vi "Handle String Data.vi"(7 "Source ID":u32, 8 "StringData":T1, 9 "Sequence":u32, 10 "ChannelService":refnum<class "ChannelService.lvclass">, 11 "Subscription Loop Data in":T2) -> (0 "error out":errorcluster, 3 "Subscription Loop Data":T2)   [LabVIEW 2020, in "Vecto.lvlib" / "RemoteDataService.lvclass"]
uses:
  RemoteDataService.lvclass
  Subscription Loop Data.ctl
  Subscription Group Info.ctl
  Group/Group.lvclass
  SubscribedDataHandler/SubscribedDataHandler.lvclass
  proto/StringData/Data.ctl
  ChannelService/ChannelService.lvclass
  <vilib>/Utility/miscctls.llb/LVMapReplaceAction.ctl
  Group STR/Group STR.lvclass
  C:/dev/lv20CE/relink/lv-vecto/Vecto/Group/Group.lvclass
  Vecto.lvlib
  proto/StringData/StringData.lvlib
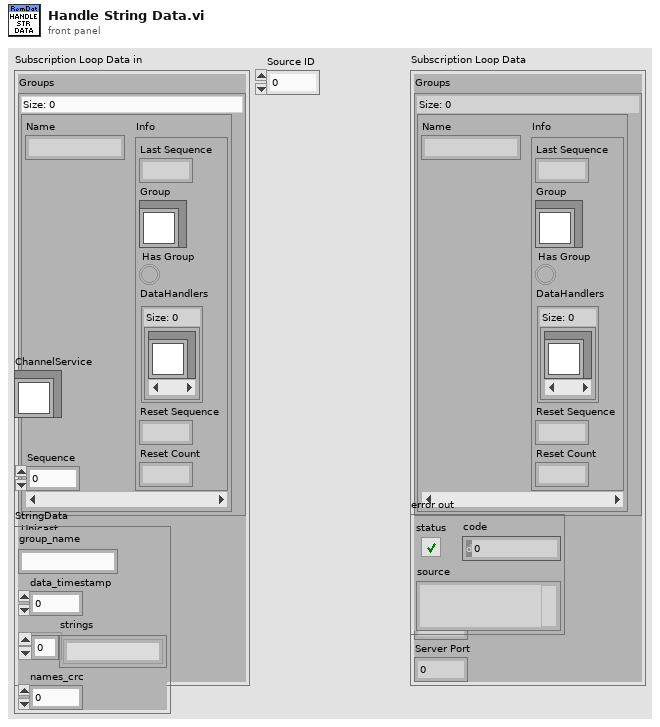
[diagram p1: front panel]
types:
  T1 = typedef "StringData.lvlib/Data.ctl" = cluster{"group_name":string, "data_timestamp":i64, "strings":string[], "names_crc":u32}
  T2 = typedef "Vecto.lvlib/RemoteDataService.lvclass/Subscription Loop Data.ctl" = cluster{"Groups":map{string, T3}, "Unicast":bool, "Last Unicast HB":dbl, "Server IP":u32, "Server Port":u16}
  T3 = typedef "Vecto.lvlib/RemoteDataService.lvclass/Subscription Group Info.ctl" = cluster{"Last Sequence":u32, "Group":refnum<class "Group.lvclass">, "Has Group":bool, "DataHandlers":set{refnum<class "SubscribedDataHandler.lvclass">}, "Reset Sequence":u32, "Reset Count":u32}
  T4 = typedef "LVMapReplaceAction.ctl" = enum32{"Modify Entry only if found", "Add or Modify Entry", "Delete Entry"}
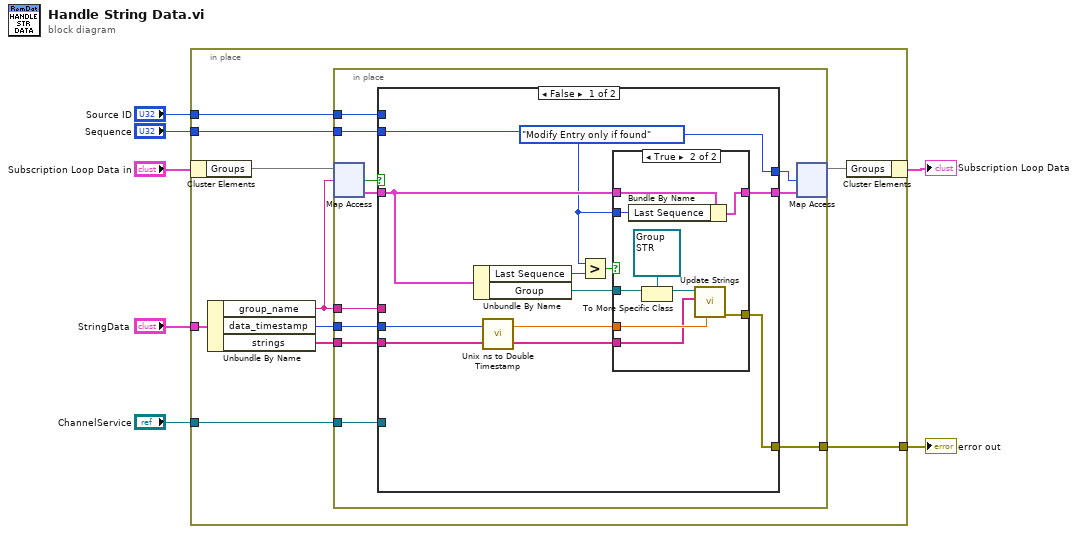
[diagram p0: block diagram]
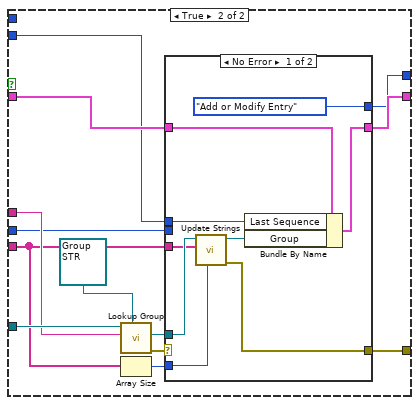
[diagram p3: hidden frame]
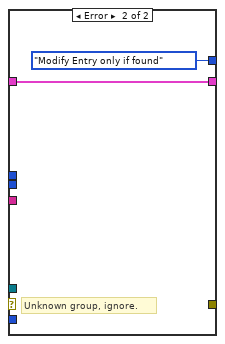
[diagram p4: hidden frame]
diagram:
  n1 = in-place {
    in-place-border: "StringData" -> [w8]
    in-place-border: "ChannelService" -> [w16]
    in-place-border: "Sequence" -> [w12]
    in-place-border: "Source ID" -> [w11]
    in-place-border: [w9] -> w2
    n2 = in-place-cluster #1("Subscription Loop Data in") -> ("Groups"=w17:map{string, T3})
    n3 = Unbundle By Name(w8) -> ("group_name"=w15:string, "data_timestamp"=w13:i64, "strings"=w14:string[])
    n4 = in-place {
      in-place-border: w16 -> [w26]
      in-place-border: w15 -> [w25]
      in-place-border: w14 -> [w24]
      in-place-border: w13 -> [w23]
      in-place-border: w12 -> [w22]
      in-place-border: w11 -> [w21]
      in-place-border: [w19] -> w9
      n5 = in-place-map #2(w17, w15) -> (w27:T3, w28:bool)  [unwired: 1 in]
      n6 = case shown="False" w28 {
        tunnel: w27 -> [w34 w57]
        tunnel: w26 -> [_ w62]
        tunnel: w25 -> [_ w60]
        tunnel: w24 -> [w35 w54]
        tunnel: w23 -> [w36 w55]
        tunnel: w22 -> [w32 w56]
        tunnel: w21 -> [_ _]
        tunnel: [w33 w53] -> w20
        tunnel: [w31 w52] -> w19
        tunnel: [LVMapReplaceAction."Modify Entry only if found" ("action") w51] -> w18
        frame False {
          n7 = Unbundle By Name(w34) -> ("Last Sequence"=w39:u32, "Group"=w38:refnum<class "Group.lvclass">)
          n8 = call "Unix ns to Double Timestamp.vi"("unix ns"=w36) -> ("Timestamp"=w29:dbl)  [unwired: 2 in]
          n9 = Greater?(x=w32, y=w39) -> (0:w37:bool)
          n10 = case shown="True" w37 {
            tunnel: w38 -> [_ w49]
            tunnel: w29 -> [_ w48]
            tunnel: w35 -> [_ w41]
            tunnel: w34 -> [w40 w47]
            tunnel: [w40 w45] -> w33
            tunnel: w32 -> [_ w46]
            tunnel: [_ w44] -> w31
            frame False {
              # "Older data, ignore"
            }
            frame True {
              n11 = Bundle By Name(cluster=w47, "Last Sequence"=w46) -> (w45:T3)
              n12 = To More Specific Class(target class=refnum<class "Group STR.lvclass"> refnum ("StringGroup in"), reference=w49) -> (specific class reference=w43:refnum<class "Group STR.lvclass">)  [unwired: 1 in, 1 out]
              n13 = call "Update Strings.vi"("Timestamp (Now)"=w48, "Strings"=w41, "StringGroup in"=w43) -> ("error out"=w44:errorcluster)  [unwired: 7 in, 1 out]
            }
          }
        }
        frame True {
          n14 = call "Lookup Group.vi"("Group Type (Abstract)"=refnum<class "Group STR.lvclass"> refnum ("Vecto.lvlib:StringGroup.lvclass"), "Group Name"=w60, "ChannelService in"=w62) -> ("error out"=w61:errorcluster, "Group"=w59:refnum<class "Group STR.lvclass">)  [unwired: 6 in, 1 out]
          n15 = Array Size(array=w54) -> (size(s)=w58:i32)
          n16 = case shown="No Error" w61 {
            tunnel: w59 -> [w65 _]
            tunnel: w58 -> [w64 _]
            tunnel: w57 -> [w71 w72]
            tunnel: w56 -> [w70 _]
            tunnel: w55 -> [_ _]
            tunnel: w54 -> [w63 _]
            tunnel: [w69 w72] -> w53
            tunnel: [w68 _] -> w52
            tunnel: [LVMapReplaceAction."Add or Modify Entry" ("action") LVMapReplaceAction."Modify Entry only if found" ("action")] -> w51
            frame No Error {
              n17 = call "Update Strings.vi"("Timestamp (Now)"=w64, "Strings"=w63, "StringGroup in"=w65) -> ("error out"=w68:errorcluster, "StringGroup out"=w67:refnum<class "Group STR.lvclass">)  [unwired: 7 in]
              n18 = Bundle By Name(cluster=w71, "Last Sequence"=w70, "Group"=w67) -> (w69:T3)
            }
            frame Error {
              # "Unknown group, ignore."
            }
          }
        }
      }
      n19 = in-place-map #2(w20, w18) -> (w10:map{string, T3})  [unwired: 2 out]
    }
    n20 = in-place-cluster #1("Groups"=w10) -> (→"Subscription Loop Data":T2)
  }
  "error out" <- w2
